vi "Set Test State.vi"(8 "error in":errorcluster, 11 "IsTestRunning":bool) -> (0 "error out":errorcluster)   [LabVIEW 2020, in "FlexLoggerTagHelpers.lvlib"]
uses:
  FlexLoggerTagHelpers.lvlib
  <vilib>/Skyline/Tag/Shared/typedefs/DataType.ctl
  System Tags.ctl
  <vilib>/Skyline/Tag/Wrapper/Wrapper AMQP_class/Open Tag AMQP.vi
  <vilib>/Skyline/Tag/Wrapper/Wrapper_class/Write Tag (Boolean).vi
  <vilib>/Skyline/Tag/Wrapper/Wrapper_class/Close Tag (Single).vi
  <vilib>/Skyline/Tag/Wrapper/Wrapper_class/NI Skyline Tag.lvclass
  <vilib>/Skyline/Tag/Shared/NI Skyline Tag.lvlib
  <vilib>/Skyline/Tag/Wrapper/Wrapper AMQP_class/NI Skyline Tag AMQP.lvclass
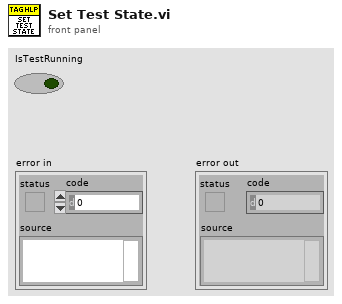
[diagram p1: front panel]
types:
  T1 = typedef "FlexLoggerTagHelpers.lvlib/System Tags.ctl" = enum16{"LastTestStart", "IsTestSessionRunning"}
  T2 = typedef "NI Skyline Tag.lvlib/DataType.ctl" = enum32{"Double", "I32", "String", "Boolean", "U64", "Timestamp"}
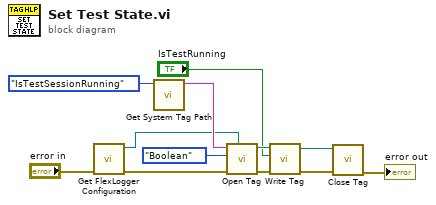
[diagram p0: block diagram]
diagram:
  n1 = call "Get FlexLogger Configuration.vi"("error in (no error)"="error in") -> ("error out"=w2:errorcluster, "Local FlexLogger Configuration"=w1:refnum<class "NI Skyline Configuration AMQP.lvclass">)  [unwired: 9 in]
  n2 = call "Get System Tag Path.vi"("sytem tag"=System_Tags."IsTestSessionRunning") -> ("tag path"=w6:string)  [unwired: 10 in]
  n3 = call-poly <vilib>:"Open Tag.vi"("configuration"=w1, "error in (no error)"=w2, "data type"=DataType."Boolean", "path"=w6) -> ("error out"=w10:errorcluster, "tag"=w11:refnum<class "NI Skyline Tag.lvclass">)  [unwired: 6 in]
  n4 = call-poly <vilib>:"Write Tag.vi"("error in (no error)"=w10, "value"="IsTestRunning", "tag in"=w11) -> ("error out"=w9:errorcluster, "tag out"=w8:refnum<class "NI Skyline Tag.lvclass">)  [unwired: 7 in]
  n5 = call-poly <vilib>:"Close Tag.vi"("error in (no error)"=w9, "tag"=w8) -> ("error out"=→"error out":errorcluster)  [unwired: 9 in]
